vi "Inheritance test.vi"   [LabVIEW 2016, in "Instrument.Oxford1820.lvclass"]
uses:
  Instrument.Oxford1820.lvclass
  <userlib>/LevyLab/Levylab Instruments/Instrument Types/Cryostat/Instrument.Cryostat.lvclass
  <userlib>/LevyLab/Levylab Instruments/SMOs/Instrument/Instrument.lvclass
  <userlib>/LevyLab/Levylab Instruments/SMOs/LevyLab/LevyLab.lvclass
  <vilib>/JKI/JKI SMO/SMO/SMO.lvclass
  C:/Program Files (x86)/National Instruments/LabVIEW 2016/vi.lib/JKI/JKI SMO/SMO/SMO.lvclass
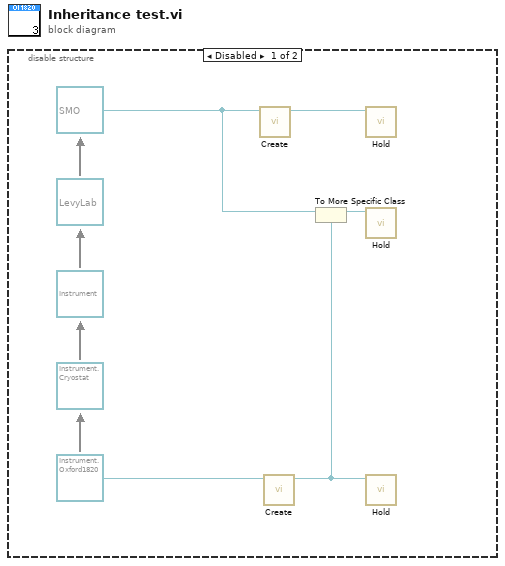
[diagram p0: block diagram]
diagram:
  n1 = disable-structure shown="Disabled" {
    frame Disabled {
      w4 = refnum<class "SMO.lvclass"> refnum ("SMO.lvclass")
      (unwired) refnum<class "LevyLab.lvclass"> refnum ("LevyLab.lvclass")
      (unwired) refnum<class "Instrument.lvclass"> refnum ("Instrument.lvclass")
      (unwired) refnum<class "Instrument.Cryostat.lvclass"> refnum ("Instrument.Cryostat.lvclass")
      n2 = call <vilib>:"Create.vi"("SMO"=w4) -> ("SMO out"=w5:refnum<class "SMO.lvclass">)  [unwired: 8 in, 2 out]
      n3 = call <vilib>:"Create.vi"("SMO"=refnum<class "Instrument.Oxford1820.lvclass"> refnum ("Instrument.Oxford1820.lvclass")) -> ("SMO out"=w1:refnum<class "Instrument.Oxford1820.lvclass">)  [unwired: 8 in, 2 out]
      n4 = To More Specific Class(target class=w1, reference=w4) -> (specific class reference=w2:refnum<class "Instrument.Oxford1820.lvclass">)  [unwired: 1 in, 1 out]
      n5 = call "Hold.vi"("Instrument.1820 in"=w5) -> ()  [unwired: 8 in, 3 out]
      n6 = call "Hold.vi"("Instrument.1820 in"=w2) -> ()  [unwired: 8 in, 3 out]
      n7 = call "Hold.vi"("Instrument.1820 in"=w1) -> ()  [unwired: 8 in, 3 out]
    }
    frame Enabled {
    }
  }
